vi "Create ID.vi"() -> (0 "id":string)   [LabVIEW 2019, in "JSON-RPC.lvlib"]
uses:
  JSON-RPC.lvlib
  <userlib>/_OpenG.lib/numeric/numeric.llb/Random Number Within Range - I32__ogtk.vi
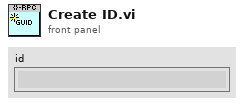
[diagram p1: front panel]
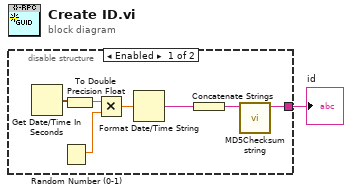
[diagram p0: block diagram]
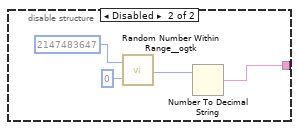
[diagram p2: hidden frame]
diagram:
  n1 = disable-structure shown="Enabled" {
    disable-tunnel: [w2 w9] -> w1
    frame Enabled {
      n2 = Get Date/Time In Seconds() -> (seconds since 1Jan1904=w6:timestamp)
      n3 = Random Number (0-1)() -> (number: 0 to 1=w3:dbl)
      n4 = To Double Precision Float(number=w6) -> (double precision float=w7:dbl)
      n5 = Multiply(x=w7, y=w3) -> (x*y=w8:dbl)
      n6 = Format Date/Time String(seconds (now)=w8) -> (date/time string=w5:string)  [unwired: 2 in]
      n7 = Concatenate Strings(w5) -> (w4:string)
      n8 = call <vilib>:"MD5Checksum string.vi"("Message String"=w4) -> ("MD5 message-digest"=w2:string)  [unwired: 10 in]
    }
    frame Disabled {
      n9 = call-poly <userlib>:"Random Number Within Range__ogtk.vi"("High"=2147483647, "Low"=0) -> ("Random Number"=w12:i32)  [unwired: 3 in]
      n10 = Number To Decimal String(number=w12) -> (decimal integer string=w9:string)  [unwired: 1 in]
    }
  }
  "id" <- w1
